vi "Transfer.Get String Buffer.vi"(11 "Transfer in":refnum<class "Transfer.lvclass">) -> (2 "Buffer":refnum<class "Buffer.lvclass">, 3 "Transfer out":refnum<class "Transfer.lvclass">)   [LabVIEW 2017, in "DSF Core.lvlib" / "Transfer.lvclass"]
uses:
  Transfer.lvclass
  Buffer/Buffer.lvclass
  Transfer.lvclass/Transfer.ctl
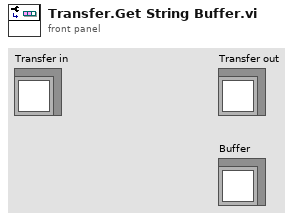
[diagram p1: front panel]
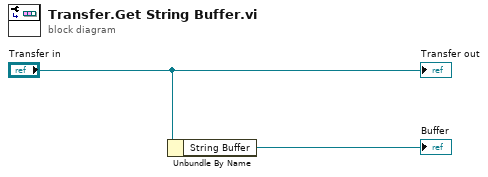
[diagram p0: block diagram]
diagram:
  n1 = Unbundle By Name("Transfer in") -> ("String Buffer"=→"Buffer":refnum<class "Buffer.lvclass">)
  "Transfer out" <- "Transfer in"
